vi "Generate Numbers without Loops.vi"(10 "Lower Limit":dbl, 11 "Upper Limit":dbl) -> (3 "Numbers":dbl[](array[numeric]))   [LabVIEW 2020]
doc: "This VI will generate Numbers within the specified LIMIT in an ascending order 1D Array without using Loops."
uses:
  <vilib>/Analysis/1siggen.llb/Ramp Pattern by Samples.vi
  00ad81d7-c4b3-46ed-ad02-d031f88f9eb0.vi
  <vilib>/Analysis/NI_AALBase.lvlib
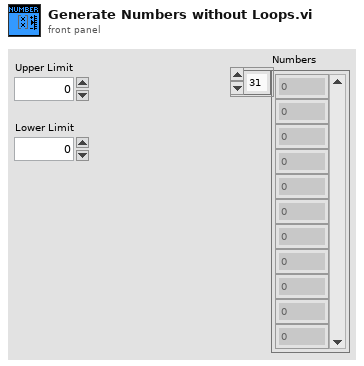
[diagram p1: front panel]
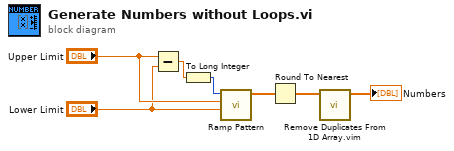
[diagram p0: block diagram]
diagram:
  n1 = Subtract(x="Upper Limit", y="Lower Limit") -> (x-y=w3:dbl)
  n2 = To Long Integer(number=w3) -> (32bit integer=w1:i32)
  n3 = call-poly <vilib>:"Ramp Pattern.vi"("start"="Lower Limit", "end"="Upper Limit", "samples"=w1) -> ("Ramp Pattern"=w6:dbl[])  [unwired: 7 in, 1 out]
  n4 = Round To Nearest(number=w6) -> (nearest integer value=w2:dbl[])
  n5 = call "Remove Duplicates From 1D Array.vim"("array"=w2) -> ("array with duplicates removed"=→"Numbers":dbl[])  [unwired: 10 in]
